vi "PH_Powermeter_BaseClass.ProcPeriodic.vi"(0 "i ref in":refnum<vi>, 3 "ms timeout (100)":i32=100, 5 "error in (no error)":errorcluster) -> (14 "i ref out":refnum<vi>, 17 "timed out":bool, 19 "error out":errorcluster)   [LabVIEW 2014, in "PH_Powermeter_BaseClass.lvlib"]
doc: "This method serves to periodically do things. In this case, it reads the current value from the powermeter. If the Start Stop - value is true, the statistic data is read out as well. Finally, these data is send to own attributes and the GUI elements."
uses:
  PH_Powermeter_BaseClass.lvlib
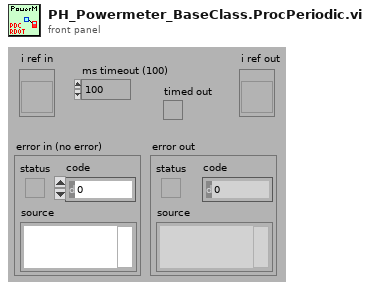
[diagram p1: front panel]
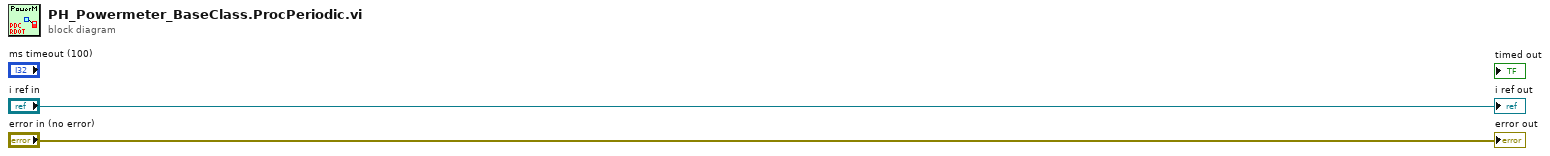
[diagram p0: block diagram]
diagram:
  "error out" <- "error in (no error)"
  "i ref out" <- "i ref in"
